vi "ResetEncoder.vi"   [LabVIEW 2014]
uses:
  <vilib>/myRIO/Instrument Drivers/Onboard IO/UART/typedef/VISA Configuration.ctl
  <vilib>/Instr/_visa.llb/VISA Configure Serial Port (Instr).vi
  <vilib>/myRIO/Express VI/Onboard IO/UART/UART Express VI.xnode
  <vilib>/myRIO/Instrument Drivers/Onboard IO/UART/UART.lvlib
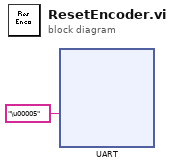
[diagram p0: block diagram]
diagram:
  n1 = xnode "UART"("Characters to Write"="\u00005") -> ()  [unwired: 1 in, 2 out]
